vi "DatabaseHand_SetSubElement.vi"(0 "Database RefNum in":T3, 1 "name":string, 2 "unit":string, 3 "value":string, 5 "enqueue? (F)":bool, 7 "Object Data In":T2, 9 "Index":i32, 11 "error in (no error)":errorcluster, 12 "type":string, 13 "permissions":string, 14 "group":string) -> (4 "Database RefNum out":T3, 10 "SubEle Out":T1, 15 "error out":errorcluster)   [LabVIEW 2016]
doc: "This VI finds the RefNum of an existing object with the input Name or creates a new object if the Name is not found or Name is unwired or an empty string.\nCopyright 2001 VI Engineering, Inc."
uses:
  DatabaseHand_RefNum.ctl
  DatabaseHand_Element.ctl
  DatabaseHan_DatabaseElement.ctl
panel:
  out "created new?":bool
  in  "DatabaseHan_DatabaseElement":T1
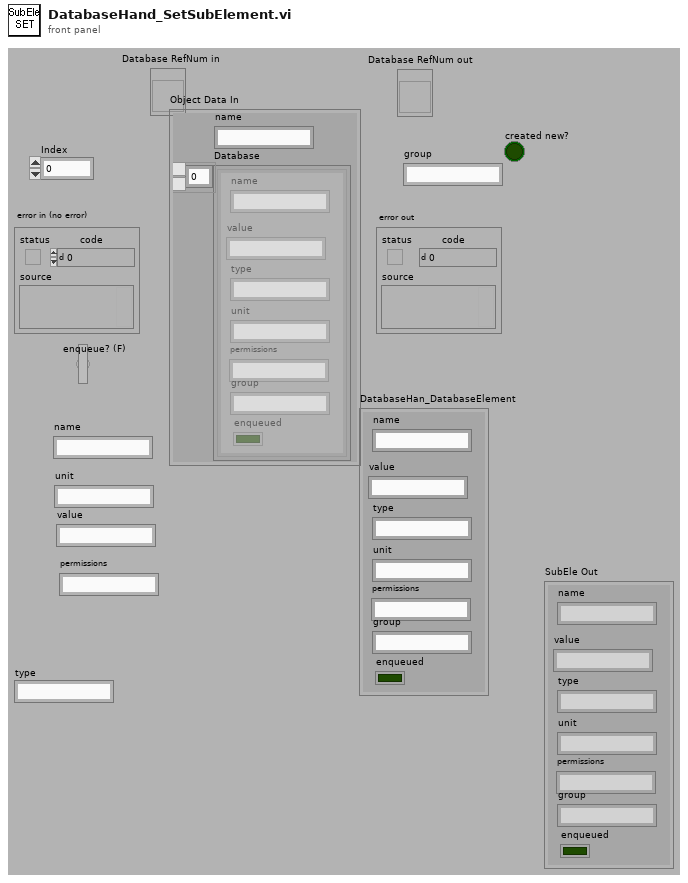
[diagram p1: front panel]
types:
  T1 = typedef "DatabaseHan_DatabaseElement.ctl" = cluster{"name":string, "value":string, "type":string, "unit":string, "permissions":string, "enqueued":bool, "group":string}
  T2 = typedef "DatabaseHand_Element.ctl" = cluster{"name":string, "Database":T1[]}
  T3 = typedef "DatabaseHand_RefNum.ctl" = refnum<vi>
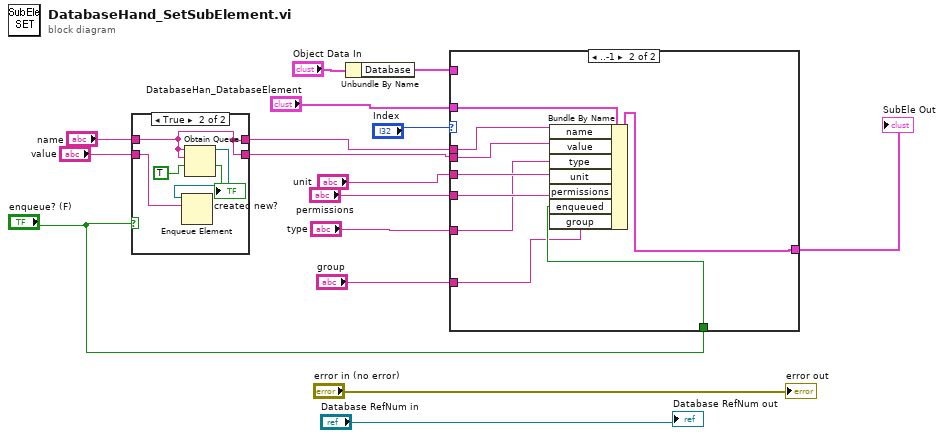
[diagram p0: block diagram]
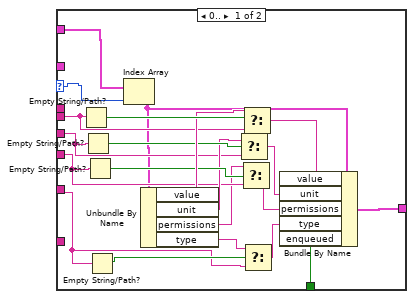
[diagram p3: hidden frame]
diagram:
  n1 = case shown="True" "enqueue? (F)" {
    tunnel: "value" -> [w18 w20]
    tunnel: [w18 w22] -> w7
    tunnel: "name" -> [w17 w22]
    tunnel: [w17 w22] -> w5
    frame False {
    }
    frame True {
      n2 = Obtain Queue(name (unnamed)=w22, element data type=w22, create if not found? (T)=TRUE ("return existing (F)")) -> (queue out=w21:refnum<queue>, created new?=→"created new?":bool)  [unwired: 2 in, 1 out]
      n3 = Enqueue Element(queue=w21, element=w20) -> ()  [unwired: 1 in, 4 out]
    }
  }
  n4 = Unbundle By Name("Object Data In") -> ("Database"=w13:T1[])
  n5 = case shown="..-1" "Index" {
    selector: "Index" -> [w43 _]
    tunnel: w13 -> [w44 _]
    tunnel: "DatabaseHan_DatabaseElement" -> [_ w53]
    tunnel: w5 -> [_ w52]
    tunnel: w7 -> [w40 w51]
    tunnel: "unit" -> [w35 w50]
    tunnel: "permissions" -> [w34 w49]
    tunnel: "type" -> [w28 w48]
    tunnel: "enqueue? (F)" -> [w26 w47]
    tunnel: "group" -> [_ w46]
    tunnel: [w24 w45] -> w2
    frame 0.. {
      n6 = Empty String/Path?(string/path=w40) -> (empty?=w42:bool)
      n7 = Empty String/Path?(string/path=w35) -> (empty?=w38:bool)
      n8 = Empty String/Path?(string/path=w34) -> (empty?=w37:bool)
      n9 = Empty String/Path?(string/path=w28) -> (empty?=w30:bool)
      n10 = Index Array(array=w44, index=w43) -> (element=w25:T1)
      n11 = Unbundle By Name(w25) -> ("value"=w41:string, "unit"=w36:string, "permissions"=w33:string, "type"=w29:string)
      n12 = Select(t=w36, s=w38, f=w35) -> (s? t:f=w32:string)
      n13 = Select(t=w33, s=w37, f=w34) -> (s? t:f=w31:string)
      n14 = Select(t=w41, s=w42, f=w40) -> (s? t:f=w39:string)
      n15 = Select(t=w29, s=w30, f=w28) -> (s? t:f=w27:string)
      n16 = Bundle By Name(cluster=w25, "value"=w39, "unit"=w32, "permissions"=w31, "type"=w27, "enqueued"=w26) -> (w24:T1)
    }
    frame ..-1 {
      n17 = Bundle By Name(cluster=w53, "name"=w52, "value"=w51, "type"=w48, "unit"=w50, "permissions"=w49, "enqueued"=w47, "group"=w46) -> (w45:T1)
    }
  }
  "SubEle Out" <- w2
  "error out" <- "error in (no error)"
  "Database RefNum out" <- "Database RefNum in"
